vi "IsInput.vi"(6 "error in":errorcluster, 9 "Tunnel in":refnum<class "Tunnel.lvclass">) -> (0 "error out":errorcluster, 3 "Tunnel out":refnum<class "Tunnel.lvclass">, 4 "Input":bool)   [LabVIEW 2014, in "Raspberry Pi Compatible Compiler for LabVIEW.lvlib" / "Tunnel.lvclass"]
uses:
  Tunnel.lvclass
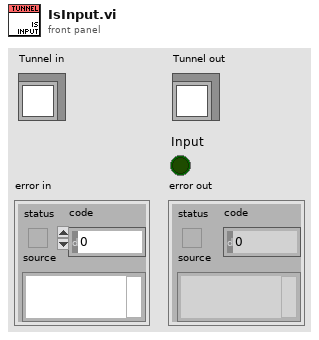
[diagram p1: front panel]
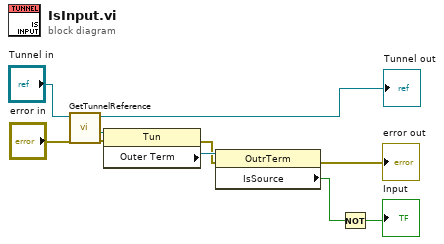
[diagram p0: block diagram]
diagram:
  n1 = call "GetTunnelReference.vi"("error in"="error in", "Tunnel in"="Tunnel in") -> ("error out"=w5:errorcluster, "reference out"=w4:refnum<vi>, "Tunnel out"=→"Tunnel out":refnum<class "Tunnel.lvclass">)  [unwired: 7 in]
  n2 = property class="Tun"(reference=w4, error in=w5) -> (error out=w9:errorcluster, "Outer Term"=w10:refnum<vi>)  [unwired: 1 out]
  n3 = property class="OutrTerm"(reference=w10, error in=w9) -> (error out=→"error out":errorcluster, "IsSource"=w2:bool)  [unwired: 1 out]
  n4 = Not(x=w2) -> (.not. x?=→"Input":bool)
